vi "Continue Sweep Waveform.vi"(8 "error in (no error)":errorcluster, 9 "Sweep Index":i32, 10 "Waveforms in":waveform(dbl)[](array[waveform]), 11 "Generator in":refnum<class "Generator.lvclass">) -> (0 "error out":errorcluster, 2 "Waveforms out":waveform(dbl)[](array[waveform]), 3 "Generator in":refnum<class "Generator.lvclass">)   [LabVIEW 2019, in "Generator.lvclass"]
uses:
  Generator.lvclass
  <vilib>/ErrorRing/Error Ring.xnode
  <vilib>/Analysis/NI_AALBase.lvlib
  Instrument.DAQ/Typedefs/Sweep.Pattern--Enum.ctl
  Instrument.DAQ/Instrument.DAQ.lvclass
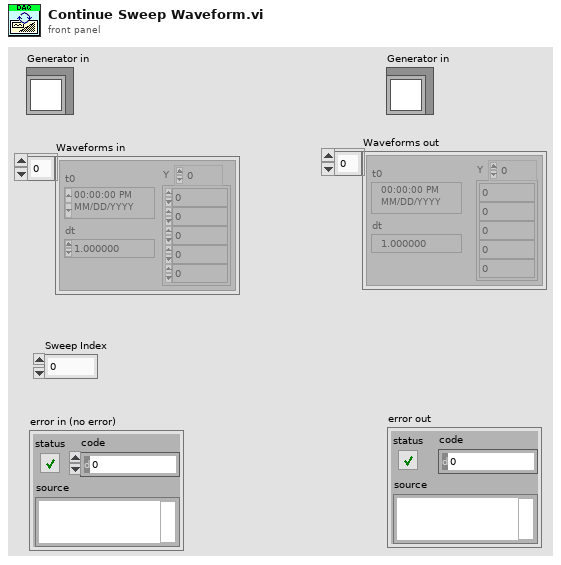
[diagram p1: front panel]
types:
  T1 = typedef "Instrument.Lockin.lvlib/Instrument.DAQ.lvclass/Sweep.Pattern--Enum.ctl" = enum16{"Ramp /", "Ramp /\\", "Smooth Ramp _/", "Smooth Ramp _/\\_", "Table"}
  T2 = typedef "Instrument.Lockin.lvlib/Instrument.DAQ.lvclass/AO.Channel--Cluster--Array.ctl" = T3[]
  T3 = typedef "Instrument.Lockin.lvlib/Instrument.DAQ.lvclass/AO.Channel--Cluster.ctl" = cluster{"Enable?":bool, "Channel":i32, "Amplitude":dbl, "Offset":dbl, "Frequency":dbl, "Phase":dbl, "Function":T4, "Sweeping?":bool, "Limit AC":bool, "Limit DC?":bool}
  T4 = typedef "Instrument.Lockin.lvlib/Instrument.DAQ.lvclass/AO.Channel.Function--Enum.ctl" = enum16{"Sine", "Triangle", "Square"}
  T5 = typedef "Instrument.Lockin.lvlib/Instrument.DAQ.lvclass/Sweep.Channel--Cluster--Array.ctl" = T6[]
  T6 = typedef "Instrument.Lockin.lvlib/Instrument.DAQ.lvclass/Sweep.Channel--Cluster.ctl" = cluster{"Enable?":bool, "Channel":u16, "Start":dbl, "End":dbl, "Pattern":T1, "Table":dbl[]}
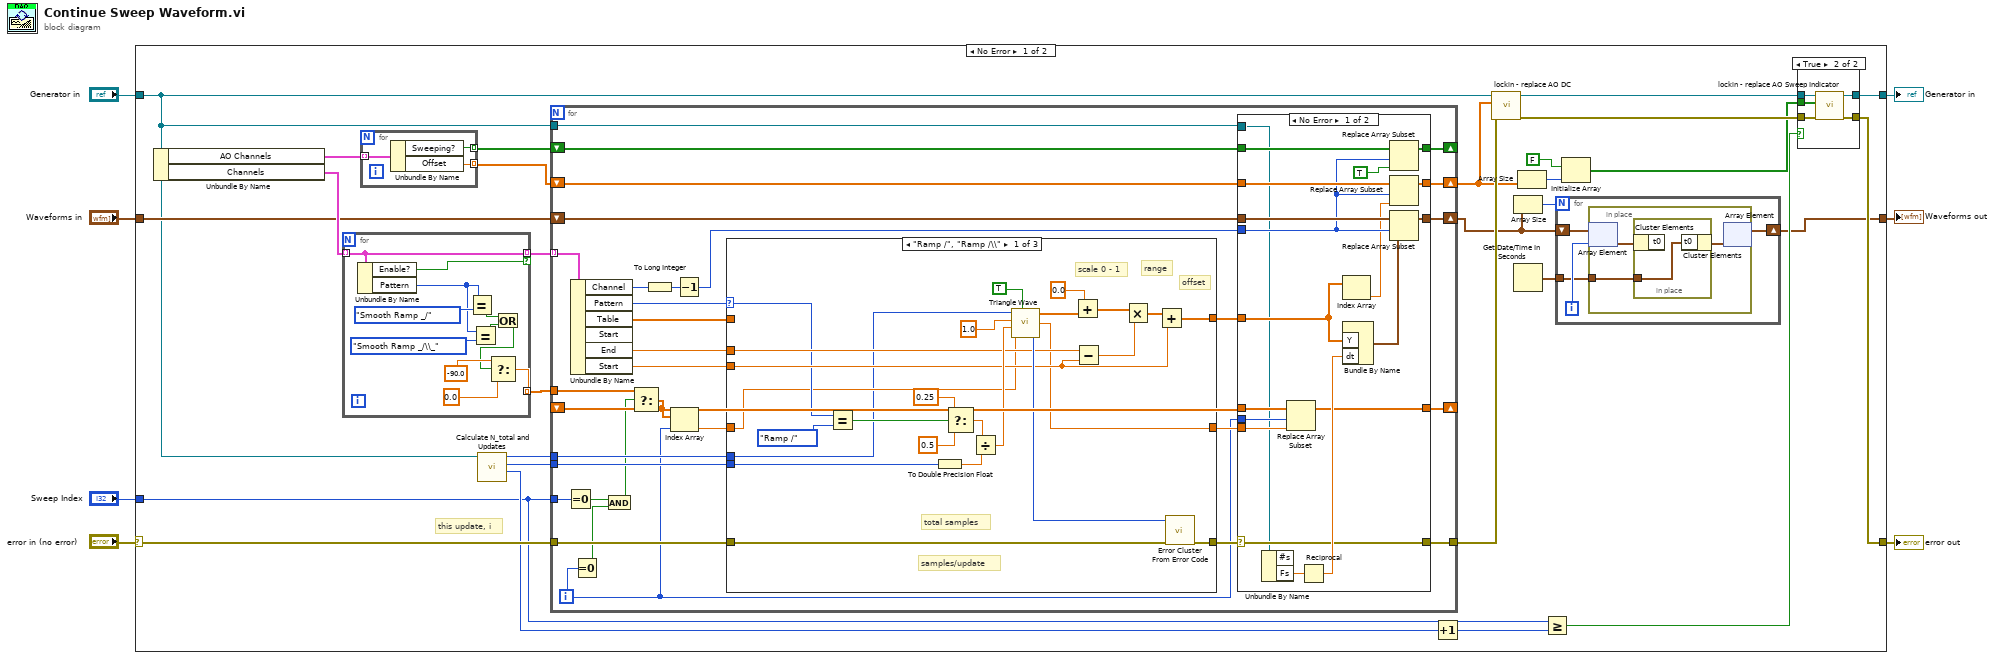
[diagram p0: block diagram]
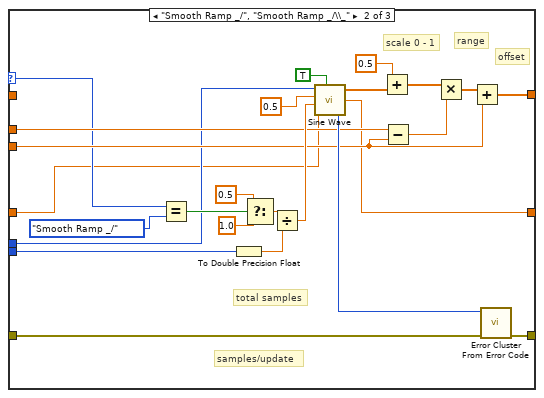
[diagram p2: hidden frame]
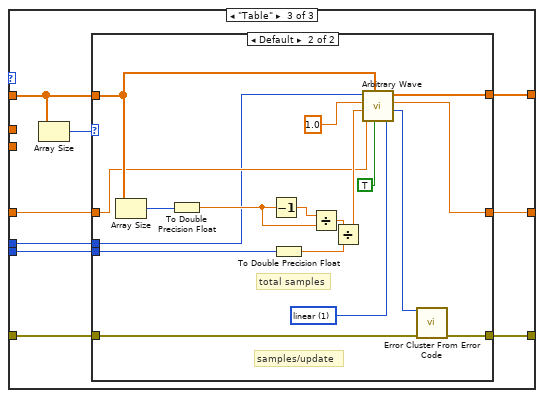
[diagram p3: hidden frame]
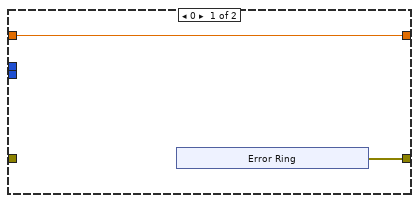
[diagram p4: hidden frame]
diagram:
  n1 = case shown="No Error" "error in (no error)" {
    selector: "error in (no error)" -> [w31 w206]
    tunnel: [w24 w206] -> w6
    tunnel: "Generator in" -> [w15 w205]
    tunnel: [w25 w205] -> w4
    tunnel: "Waveforms in" -> [w30 _]
    tunnel: [w8 _] -> w2
    tunnel: "Sweep Index" -> [w18 _]
    frame No Error {
      # "this update, i"
      n2 = Unbundle By Name(w15) -> ("AO Channels"=w32:T2, "Channels"=w35:T5)
      n3 = for {
        tunnel: w35 -> [w197] mode=indexing
        tunnel: [w197] -> w13 mode=indexing if=w196
        tunnel: [w187] -> w12 mode=indexing
        n4 = Unbundle By Name(w197) -> ("Enable?"=w196:bool, "Pattern"=w194:T1)
        n5 = Equal?(x=w194, y=Sweep.Pattern--Enum."Smooth Ramp _/" ("Pattern")) -> (x = y?=w192:bool)
        n6 = Equal?(x=w194, y=Sweep.Pattern--Enum."Smooth Ramp _/\\_" ("Pattern")) -> (x = y?=w191:bool)
        n7 = Or(x=w192, y=w191) -> (x .or. y?=w188:bool)
        n8 = Select(t=-90.0 ("phase in"), s=w188, f=0.0 ("element")) -> (s? t:f=w187:dbl)
      }
      n9 = for {
        tunnel: [w186] -> w33 mode=indexing
        tunnel: [w185] -> w34 mode=indexing
        tunnel: w32 -> [w184] mode=indexing
        n10 = Unbundle By Name(w184) -> ("Sweeping?"=w185:bool, "Offset"=w186:dbl)
      }
      n11 = call "Calculate N_total and Updates.vi"("Generator in"=w15) -> ("Updates"=w19:i32, "Total Samples"=w14:i32, "Samples/Update"=w16:i32)  [unwired: 8 in]
      n12 = for {
        tunnel: w13 -> [w60] mode=indexing
        shift-right: [w71] -> _
        shift-left: w34 -> [w70]
        shift-right: [w68] -> w20
        shift-left: w33 -> [w69]
        shift-right: [w66] -> w9
        shift-left: w30 -> [w67]
        tunnel: w31 -> [w75]
        tunnel: [w59] -> w23
        tunnel: w18 -> [w54]
        shift-right: [w56] -> _
        shift-left: _ -> [w51]
        tunnel: w12 -> [w53]
        tunnel: w16 -> [w50]
        tunnel: w15 -> [w49]
        tunnel: w14 -> [w48]
        i -> [w47]
        n13 = Equal To 0?(x=w54) -> (x = 0?=w46:bool)
        n14 = Unbundle By Name(w60) -> ("Channel"=w64:u16, "Pattern"=w73:T1, "Table"=w74:dbl[], "End"=w72:dbl, "Start"=w62:dbl)  [unwired: 1 out]
        n15 = Equal To 0?(x=w47) -> (x = 0?=w45:bool)
        n16 = And(x=w46, y=w45) -> (x .and. y?=w44:bool)
        n17 = Select(t=w53, s=w44, f=w51) -> (s? t:f=w52:dbl[])
        n18 = To Long Integer(number=w64) -> (32bit integer=w65:i32)
        n19 = Index Array(array=w52, index=w47) -> (element=w55:dbl)
        n20 = Decrement(x=w65) -> (x-1=w63:i32)
        n21 = case shown="\"Ramp /\", \"Ramp /\\\\\"" w73 {
          selector: w73 -> [w81 w107 _]
          tunnel: w72 -> [w89 w114 _]
          tunnel: [w92 w117 w132] -> w61
          tunnel: [w99 w124 w133] -> w58
          tunnel: w75 -> [w100 w125 w134]
          tunnel: w74 -> [_ _ w130]
          tunnel: w62 -> [w87 w112 _]
          tunnel: [w79 w106 w129] -> w57
          tunnel: w55 -> [w80 w102 w128]
          tunnel: w50 -> [w78 w104 w127]
          tunnel: w48 -> [w77 w103 w126]
          frame "Ramp /", "Ramp /\\" {
            # "range"
            # "total samples"
            # "samples/update"
            # "offset"
            # "scale 0 - 1"
            n22 = Equal?(x=w81, y=Sweep.Pattern--Enum."Ramp /" ("Pattern")) -> (x = y?=w83:bool)
            n23 = To Double Precision Float(number=w77) -> (double precision float=w90:dbl)
            n24 = Select(t=0.25, s=w83, f=0.5) -> (s? t:f=w84:dbl)
            n25 = Divide(x=w84, y=w90) -> (x/y=w91:dbl)
            n26 = call <vilib>:"Triangle Wave.vi"("samples"=w78, "amplitude"=1.0, "frequency"=w91, "phase in"=w80, "reset phase"=TRUE) -> ("triangle wave"=w93:dbl[], "phase out"=w79:dbl, "error"=w94:i32)
            n27 = Add(x=0.0 ("cycles 2"), y=w93) -> (x+y=w97:dbl[])
            n28 = Subtract(x=w89, y=w87) -> (x-y=w88:dbl)
            n29 = Multiply(x=w97, y=w88) -> (x*y=w96:dbl[])
            n30 = Add(x=w96, y=w87) -> (x+y=w92:dbl[])
            n31 = call <vilib>:"Error Cluster From Error Code.vi"("error in (no error)"=w100, "error code (0)"=w94) -> ("error out"=w99:errorcluster)  [unwired: 7 in]
          }
          frame "Smooth Ramp _/", "Smooth Ramp _/\\_" {
            # "range"
            # "total samples"
            # "samples/update"
            # "offset"
            # "scale 0 - 1"
            n32 = Equal?(x=w107, y=Sweep.Pattern--Enum."Smooth Ramp _/" ("Pattern")) -> (x = y?=w108:bool)
            n33 = To Double Precision Float(number=w103) -> (double precision float=w115:dbl)
            n34 = Select(t=0.5, s=w108, f=1.0) -> (s? t:f=w109:dbl)
            n35 = Divide(x=w109, y=w115) -> (x/y=w116:dbl)
            n36 = call <vilib>:"Sine Wave.vi"("samples"=w104, "amplitude"=0.5, "frequency"=w116, "phase in"=w102, "reset phase"=TRUE) -> ("sine wave"=w118:dbl[], "phase out"=w106:dbl, "error"=w119:i32)
            n37 = Add(x=0.5 ("cycles 2"), y=w118) -> (x+y=w122:dbl[])
            n38 = Subtract(x=w114, y=w112) -> (x-y=w113:dbl)
            n39 = Multiply(x=w122, y=w113) -> (x*y=w121:dbl[])
            n40 = Add(x=w121, y=w112) -> (x+y=w117:dbl[])
            n41 = call <vilib>:"Error Cluster From Error Code.vi"("error in (no error)"=w125, "error code (0)"=w119) -> ("error out"=w124:errorcluster)  [unwired: 7 in]
          }
          frame "Table" {
            n42 = Array Size(array=w130) -> (size(s)=w131:i32)
            n43 = case shown="Default" w131 {
              tunnel: w134 -> [_ w159]
              tunnel: [w136 w158] -> w133
              tunnel: w130 -> [_ w153]
              tunnel: [_ w155] -> w132
              tunnel: [w135 w146] -> w129
              tunnel: w128 -> [w135 w145]
              tunnel: w127 -> [_ w144]
              tunnel: w126 -> [_ w143]
              frame 0 {
                n44 = xnode "Error Ring"() -> ("error out"=w136:errorcluster)
              }
              frame Default {
                w154 = 1 items=["none", "linear"] ("interpolation")
                # "total samples"
                # "samples/update"
                n45 = Array Size(array=w153) -> (size(s)=w152:i32)
                n46 = To Double Precision Float(number=w152) -> (double precision float=w147:dbl)
                n47 = Decrement(x=w147) -> (x-1=w148:dbl)
                n48 = To Double Precision Float(number=w143) -> (double precision float=w151:dbl)
                n49 = Divide(x=w148, y=w147) -> (x/y=w150:dbl)
                n50 = Divide(x=w150, y=w151) -> (x/y=w149:dbl)
                n51 = call <vilib>:"Arbitrary Wave.vi"("interpolation"=w154, "reset phase"=TRUE, "Wave Table"=w153, "phase in"=w145, "frequency"=w149, "amplitude"=1.0, "samples"=w144) -> ("error"=w156:i32, "phase out"=w146:dbl, "arbitrary wave"=w155:dbl[])
                n52 = call <vilib>:"Error Cluster From Error Code.vi"("error in (no error)"=w159, "error code (0)"=w156) -> ("error out"=w158:errorcluster)  [unwired: 7 in]
              }
            }
          }
        }
        n53 = case shown="No Error" w58 {
          selector: w58 -> [w165 w183]
          tunnel: [w177 w180] -> w71
          tunnel: w70 -> [w176 w180]
          tunnel: w69 -> [w175 w181]
          tunnel: [w174 w181] -> w68
          tunnel: w67 -> [w173 w182]
          tunnel: [w172 w182] -> w66
          tunnel: w63 -> [w171 _]
          tunnel: w61 -> [w166 _]
          tunnel: [w165 w183] -> w59
          tunnel: w57 -> [w164 _]
          tunnel: w47 -> [w163 _]
          tunnel: w52 -> [w162 w179]
          tunnel: [w161 w179] -> w56
          tunnel: w49 -> [w160 _]
          frame No Error {
            n54 = Unbundle By Name(w160) -> ("Fs"=w168:dbl)  [unwired: 1 out]
            n55 = Replace Array Subset(array=w162, new element=w164, index=w163) -> (w161:dbl[])
            n56 = Reciprocal(x=w168) -> (1/x=w167:dbl)
            n57 = Index Array(array=w166) -> (element=w170:dbl)  [unwired: 1 in]
            n58 = Bundle By Name("Y"=w166, "dt"=w167) -> (w169:waveform(dbl))  [unwired: 1 in]
            n59 = Replace Array Subset(array=w176, new element=TRUE ("new element/subarray"), index=w171) -> (w177:bool[])
            n60 = Replace Array Subset(array=w175, new element=w170, index=w171) -> (w174:dbl[])
            n61 = Replace Array Subset(array=w173, new element=w169, index=w171) -> (w172:waveform(dbl)[])
          }
          frame Error {
          }
        }
      }
      n62 = Increment(x=w19) -> (x+1=w17:i32)
      n63 = call "lockin - replace AO DC.vi"("error in (no error)"=w23, "AO.DC (V)"=w20, "Generator in"=w15) -> ("error out"=w26:errorcluster, "Generator out"=w28:refnum<class "Generator.lvclass">)  [unwired: 7 in]
      n64 = Array Size(array=w9) -> (size(s)=w10:i32)
      n65 = Get Date/Time In Seconds() -> (seconds since 1Jan1904=w11:timestamp)
      n66 = Array Size(array=w20) -> (size(s)=w27:i32)
      n67 = Greater Or Equal?(x=w18, y=w17) -> (x >= y?=w21:bool)
      n68 = for {
        N: w10 -> [_]
        shift-right: [w38] -> w8
        shift-left: w9 -> [w39]
        tunnel: w11 -> [w36]
        i -> [w37]
        n69 = in-place {
          in-place-border: w36 -> [w41]
          n70 = in-place-array #1(w39, w37) -> (w42:waveform(dbl))
          n71 = in-place {
            in-place-border: w41 -> [w43]
            n72 = in-place-cluster #2(w42) -> ()  [unwired: 1 out]
            n73 = in-place-cluster #2("t0"=w43) -> (w40:waveform(dbl))
          }
          n74 = in-place-array #1(w40) -> (w38:waveform(dbl)[])  [unwired: 1 out]
        }
      }
      n75 = Initialize Array(FALSE, w27) -> (w22:bool[])
      n76 = case shown="True" w21 {
        tunnel: w28 -> [w199 w204]
        tunnel: [w199 w203] -> w25
        tunnel: w26 -> [w198 w202]
        tunnel: [w198 w201] -> w24
        tunnel: w22 -> [_ w200]
        frame False {
        }
        frame True {
          n77 = call "lockin - replace AO Sweep Indicator.vi"("error in (no error)"=w202, "Channels: AO.Sweeping?"=w200, "Generator in"=w204) -> ("error out"=w201:errorcluster, "Generator out"=w203:refnum<class "Generator.lvclass">)  [unwired: 7 in]
        }
      }
    }
    frame Error {
    }
  }
  "error out" <- w6
  "Generator in" <- w4
  "Waveforms out" <- w2
